vi "Write CS++Factory.vi"(8 "Error In":errorcluster, 10 "CS++Factory.lvclass":refnum<class "CS++Factory.lvclass">, 11 "CS++RTRootActor in":refnum<class "CS++RTRootActor.lvclass">) -> (0 "Error Out":errorcluster, 3 "CS++RTRootActor out":refnum<class "CS++RTRootActor.lvclass">)   [LabVIEW 2015, in "CS++RTRoot.lvlib" / "CS++RTRootActor.lvclass"]
doc: "Write Factory to attribute."
uses:
  CS++RTRootActor.lvclass
  CSPP_Core/Classes/CS++BaseClasses/Factory/CS++Factory.lvclass
  CS++RTRootActor.lvclass/CS++RTRootActor.ctl
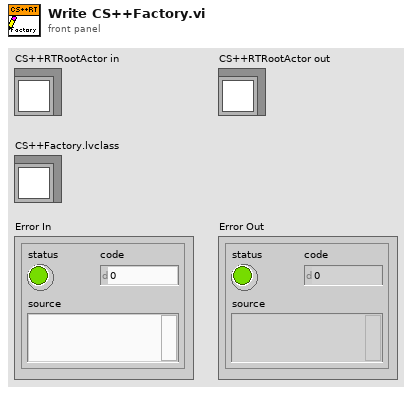
[diagram p1: front panel]
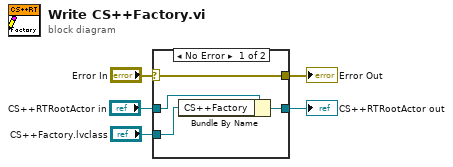
[diagram p0: block diagram]
diagram:
  n1 = case shown="No Error" "Error In" {
    selector: "Error In" -> [w9 w10]
    tunnel: [w9 w10] -> w4
    tunnel: [w7 w11] -> w2
    tunnel: "CS++RTRootActor in" -> [w8 w11]
    tunnel: "CS++Factory.lvclass" -> [w6 _]
    frame No Error {
      n2 = Bundle By Name(cluster=w8, "CS++Factory"=w6) -> (w7:refnum<class "CS++RTRootActor.lvclass">)
    }
    frame Error {
    }
  }
  "Error Out" <- w4
  "CS++RTRootActor out" <- w2
